vi "DCC Get Single Parameter.vi"(7 "Parameter IDs":T1, 8 "Error In":errorcluster, 10 "Module No":i16, 11 "DLL Path":path) -> (0 "Error Out":errorcluster, 2 "Module No":i16, 3 "DLL Path":path, 4 "New Value":sgl)   [LabVIEW 2019]
doc: "The procedure loads ‘value’ with the actual value of the requested parameter from the DLLinternal data structures of the DCC module ‘mod_no’. First two par_id values ( 0 - ACTIVE and 1 - PCI_BUS_NO) are not allowed - return error code. The par_id values are defined in dcc_def.h file as DCC_PARAMETERS_KEYWORDS.\n\nAugust 2018\nFrank Quadt & Stefan Smietana\ninfo@becker-hickl.com"
uses:
  DCC_Controls/DCC_ParameterIDs.ctl
panel:
  # "(c) 2021 Becker & Hickl GmbH\n     Al Rights Reserved."
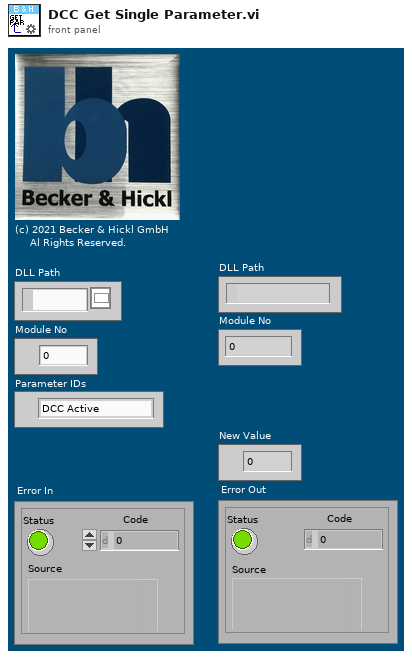
[diagram p1: front panel]
types:
  T1 = typedef "DCC_ParameterIDs.ctl" = enum16{"DCC Active", "PCI BUS No", "C1 +5 V", "C1-5 V", "C1 +12 V", "C1 Gain HV[%]", "C2 +5 V", "C2 -5 V", "C2 +12 V", "C2 Digout", "C3 Cooling", "C3 Cooling [V]", "C3 Cooling [A]", "C3 Gain HV [%]", "C3 +5 V", "C3 -5 V", "C3 +12 V"}
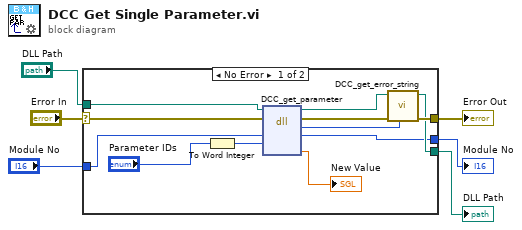
[diagram p0: block diagram]
diagram:
  n1 = case shown="No Error" "Error In" {
    selector: "Error In" -> [w18 w20]
    tunnel: [w14 w20] -> w5
    tunnel: [w13 w19] -> w4
    tunnel: "DLL Path" -> [w17 w19]
    tunnel: "Module No" -> [w12 w21]
    tunnel: [w10 w21] -> w1
    frame No Error {
      n2 = To Word Integer(number="Parameter IDs") -> (16bit integer=w8:i16)
      n3 = dll-call lib="C:/Program Files (x86)/BH/DCC/DLL/dcc64.dll" fn="DCC_get_parameter"(path in=w17, error in=w18, "ModuleNo"=w12, "ParameterID"=w8) -> (path out=w16:path, error out=w15:errorcluster, "return type"=w11:i16, "ModuleNo"=w10:i16, "NewValue"=→"New Value":sgl)  [unwired: 3 in]
      n4 = call "DCC_get_error_string.vi"("Error ID"=w11, "Error In"=w15, "DLL Path"=w16) -> ("Error Out"=w14:errorcluster, "DLL Path"=w13:path)  [unwired: 6 in, 1 out]
    }
    frame Error {
    }
  }
  "Error Out" <- w5
  "DLL Path" <- w4
  "Module No" <- w1
